vi "Simple Temperature Monitor RT Host.vi"() -> ()   [LabVIEW 2010]
uses:
  <vilib>/rvi/interface/nirviOpenFPGA/nirviOpenFPGA.xnode
  <vilib>/rvi/interface/nirviCloseFPGA/nirviCloseFPGA.xnode
  <vilib>/rvi/interface/nirviReadWriteControl/nirviReadWriteControl.xnode
  Temperature Monitor FPGA.vi
  <vilib>/userDefined/High Color/nirio_resource_hc.ctl
  NI 9211 Support Files.llb/NI 9211 Convert to Temperature (Calibrated).vi
  FPGA Bitfiles/Temperature Monito~B4_FPGA Target_Temperature Monito~96.lvbitx
  <vilib>/RVI Host/nirviSupport.llb/nirviErrorClusterFromErrorCode.vi
  <vilib>/rvi/errors/niLvFpgaWhatHappensToTopLevelVI.ctl
  <vilib>/rvi/interface/common/niFpgaNodeNameForErrorReporting.ctl
  <vilib>/rvi/errors/niLvFpgaAdjustHostInterfaceError.vi
  <vilib>/FPGAPlugInAG/cRIO-9074/niLvFpga_Close_cRIO-9074.vi
panel:
  in  "stop":bool
  in  "Sample Period (ms)":u32=500
  out "Temperature":sgl(graph)
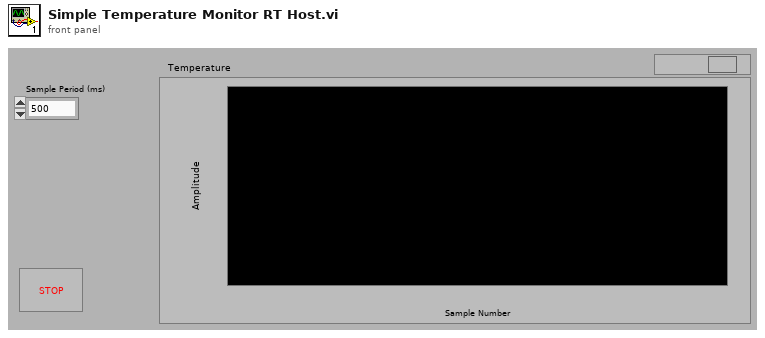
[diagram p1: front panel]
types:
  T1 = typedef "niFpgaNodeNameForErrorReporting.ctl" = enum16{"Open FPGA VI Reference", "Read/Write Control", "Invoke Method: Abort", "Invoke Method: Acknowledge IRQ", "Invoke Method: Download", "Invoke Method: FIFO.Configure", "Invoke Method: FIFO.Read", "Invoke Method: FIFO.Start", "Invoke Method: FIFO.Stop", "Invoke Method: FIFO.Write", "Invoke Method: Reset", "Invoke Method: Run", "Invoke Method: Wait on IRQ", "Close FPGA VI Reference"}
  T2 = typedef "niLvFpgaWhatHappensToTopLevelVI.ctl" = enum16{"top level VI scripted behind XNode", "top level VI inlined behind XNode"}
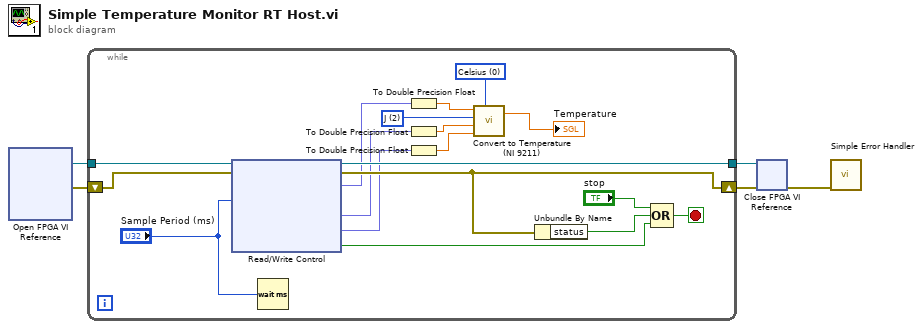
[diagram p0: block diagram]
diagram:
  n1 = xnode "Open FPGA VI Reference"() -> ("FPGA VI Reference Out"=w2:refnum<k20>, "error out"=w5:errorcluster)  [unwired: 2 in]
  n2 = while {
    shift-right: [w21] -> w3
    shift-left: w5 -> [w23]
    tunnel: w2 -> [w16]
    tunnel: [w22] -> w4
    stop <- w17 stop-if-true
    w10 = u16 0 items=["Celsius", "Fahrenheit", "Kelvin", "Rankine"] ("Temperature Units (C)")
    w9 = u16 2 items=["B", "E", "J", "K", "R", "S", "T", "N", "IC (C)", "IC (F)", "Therm."] ("ThermocoupleType")
    n3 = xnode "Read/Write Control"("FPGA VI Reference In"=w16, "error in"=w23, "Sample Period (ms)"="Sample Period (ms)") -> ("FPGA VI Reference Out"=w22:refnum<k20>, "error out"=w21:errorcluster, "Temperature"=w15:fxp<+/-,24,-2>, "CJC"=w14:fxp<+/-,24,-2>, "Autozero"=w13:fxp<+/-,24,-2>, "status"=w12:bool)
    n4 = Wait (ms)(milliseconds to wait="Sample Period (ms)") -> ()  [unwired: 1 out]
    n5 = To Double Precision Float(number=w15) -> (double precision float=w11:dbl)
    n6 = To Double Precision Float(number=w14) -> (double precision float=w8:dbl)
    n7 = To Double Precision Float(number=w13) -> (double precision float=w7:dbl)
    n8 = call-poly "Convert to Temperature (NI 9211).vi"("Temperature Units (C)"=w10, "Autozero Channel"=w7, "CJC Channel"=w8, "ThermocoupleType"=w9, "Thermocouple Channel"=w11) -> ("Linearized Temperature"=→"Temperature":sgl)  [unwired: 2 in]
    n9 = Unbundle By Name "Unbundle By Name"(w21) -> ("status"=w19:bool)
    n10 = Compound Arithmetic op=OR("stop", w19, w12) -> (w17:bool)
  }
  n11 = xnode "Close FPGA VI Reference"("FPGA VI Reference In"=w4, "error in"=w3) -> ("error out"=w1:errorcluster)
  n12 = call <vilib>:"Simple Error Handler.vi"("error in (no error)"=w1) -> ()  [unwired: 1 in, 8 out]
